vi "Delete Old Files.vi"(8 "error in (no error)":errorcluster, 9 "N Day Buffer":u32, 10 "file extension":string, 11 "location":path) -> (0 "error out":errorcluster)   [LabVIEW 2019, in "TSC Event Logger.lvlib" / "Log Sinks.lvclass"]
uses:
  Text File/Text File.lvclass/Text File.ctl
  <vilib>/Utility/miscctls.llb/LVDateTimeRec.ctl
  Log Sinks.lvclass
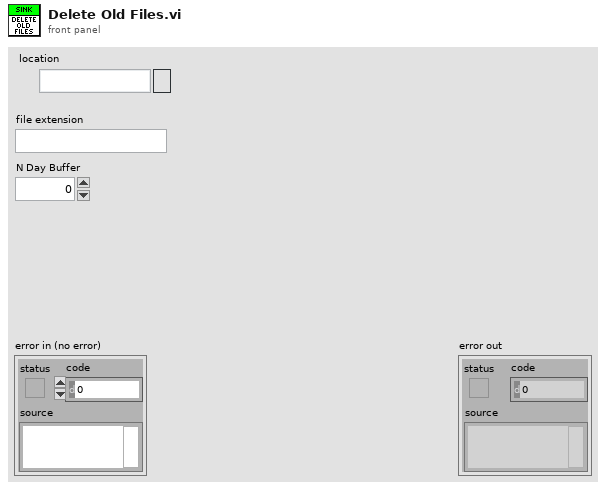
[diagram p1: front panel]
types:
  T1 = typedef "LVDateTimeRec.ctl" = cluster{"fractional second":dbl, "second":i32, "minute":i32, "hour":i32, "day of month":i32, "month":i32, "year":i32, "day of week":i32, "day of year":i32, "DST":i32}
  T2 = cluster{"Year":u16, "Month":u16, "DayOfWeek":u16, "Day":u16, "Hour":u16, "Minute":u16, "Seconds":u16, "Milliseconds":u16}
  T3 = cluster{"Year":i32, "Month":i32, "DayOfWeek":i32, "Day":i32, "Hour":i32, "Minute":i32, "Seconds":i32, "Milliseconds":i32}
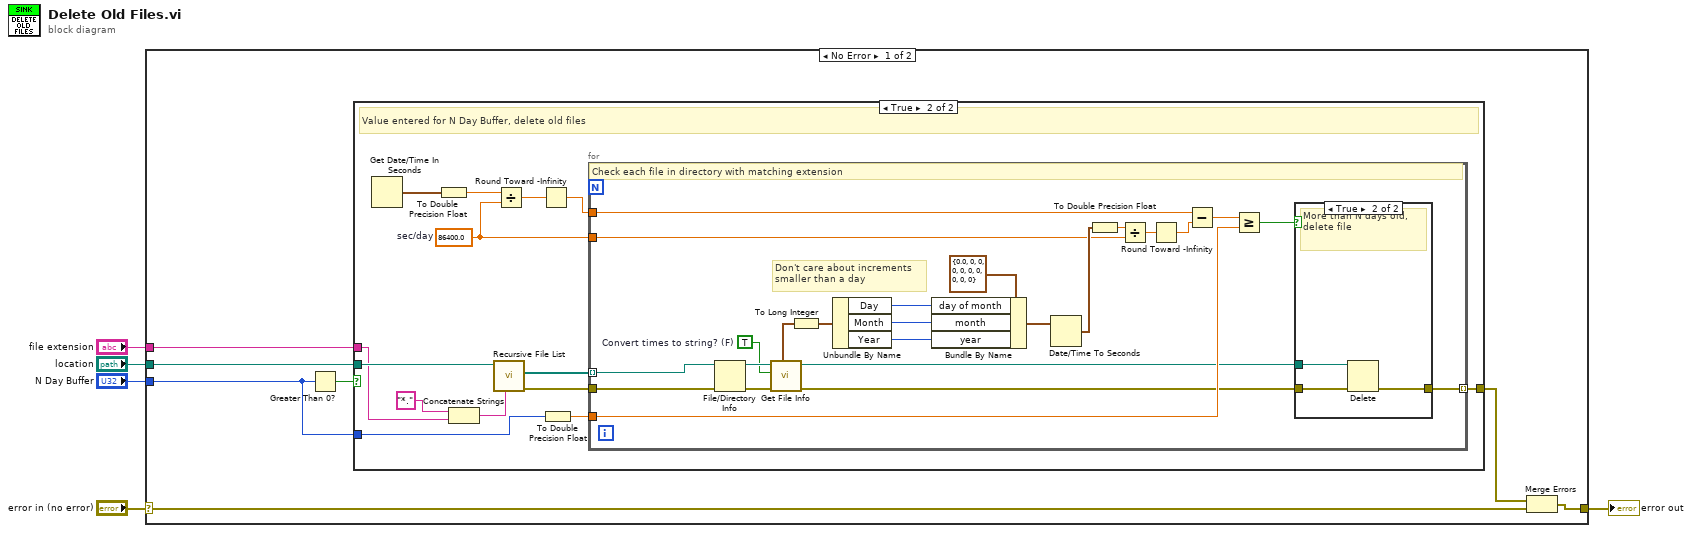
[diagram p0: block diagram]
diagram:
  n1 = case shown="No Error" "error in (no error)" {
    selector: "error in (no error)" -> [w12 w55]
    tunnel: [w10 w55] -> w4
    tunnel: "location" -> [w8 _]
    tunnel: "file extension" -> [w7 _]
    tunnel: "N Day Buffer" -> [w6 _]
    frame No Error {
      n2 = Greater Than 0?(x=w6) -> (x > 0?=w11:bool)
      n3 = case shown="True" w11 {
        tunnel: w8 -> [_ w26]
        tunnel: [_ w23] -> w9
        tunnel: w7 -> [_ w21]
        tunnel: w6 -> [_ w15]
        frame False {
        }
        frame True {
          w13 = 86400.0  # sec/day
          # "Value entered for N Day Buffer, delete old files"
          n4 = Get Date/Time In Seconds() -> (seconds since 1Jan1904=w22:timestamp)
          n5 = To Double Precision Float(number=w22) -> (double precision float=w18:dbl)
          n6 = Concatenate Strings("*." ("string"), w21) -> (w20:string)
          n7 = call <vilib>:"Recursive File List.vi"("pattern"=w20, "Folder Path"=w26) -> ("error out"=w24:errorcluster, "All Files in Dir"=w25:path[])  [unwired: 5 in, 3 out]
          n8 = Divide(x=w18, y=w13) -> (x/y=w17:dbl)
          n9 = Round Toward -Infinity(1:w17) -> (0:w16:dbl)
          n10 = To Double Precision Float(number=w15) -> (double precision float=w14:dbl)
          n11 = for {
            tunnel: w25 -> [w49] mode=indexing
            tunnel: w16 -> [w46]
            tunnel: w14 -> [w41]
            tunnel: w13 -> [w31]
            tunnel: w24 -> [w50]
            tunnel: [w30] -> w23 mode=indexing
            w40 = TRUE  # Convert times to string? (F)
            # "Don't care about increments\nsmaller than a day"
            # "Check each file in directory with matching extension"
            n12 = File/Directory Info(path=w49, error in=w50) -> (path out=w47:path, error out=w48:errorcluster)  [unwired: 5 out]
            n13 = call "Get File Info.vi"("error in (no error)"=w48, "Convert times to string? (F)"=w40, "File Path in"=w47) -> ("error out"=w29:errorcluster, "File Path out"=w28:path, "Creation Time"=w37:T2)  [unwired: 1 in, 5 out]
            n14 = To Long Integer(number=w37) -> (32bit integer=w33:T3)
            n15 = Unbundle By Name(w33) -> ("Day"=w36:i32, "Month"=w35:i32, "Year"=w34:i32)
            n16 = Bundle By Name(cluster=T1 {"fractional second"=0.0, "second"=0, "minute"=0, "hour"=0, "day of month"=0, "month"=0, "year"=0, "day of week"=0, "day of year"=0, "DST"=0} ("date time rec"), "day of month"=w36, "month"=w35, "year"=w34) -> (w38:T1)
            n17 = Date/Time To Seconds(2:w38) -> (0:w32:timestamp)  [unwired: 1 in]
            n18 = To Double Precision Float(number=w32) -> (double precision float=w44:dbl)
            n19 = Divide(x=w44, y=w31) -> (x/y=w45:dbl)
            n20 = Round Toward -Infinity(1:w45) -> (0:w43:dbl)
            n21 = Subtract(x=w46, y=w43) -> (x-y=w42:dbl)
            n22 = Greater Or Equal?(x=w42, y=w41) -> (x >= y?=w27:bool)
            n23 = case shown="True" w27 {
              tunnel: [w51 w53] -> w30
              tunnel: w29 -> [w51 w54]
              tunnel: w28 -> [_ w52]
              frame False {
              }
              frame True {
                # "More than N days old, delete file"
                n24 = Delete(path (use dialog)=w52, error in=w54) -> (error out=w53:errorcluster)  [unwired: 3 in, 2 out]
              }
            }
          }
        }
      }
      n25 = Merge Errors(w9, w12) -> (w10:errorcluster)
    }
    frame Error {
    }
  }
  "error out" <- w4
